vi "State Machine Air Heater Control.vi"() -> ()   [LabVIEW 2022 SP3]
uses:
  <vilib>/MakerHub/LINX/Public/Peripherals/Analog/Analog Read 1 Chan.vi
  <vilib>/MakerHub/LINX/Public/Peripherals/PWM/PWM Set Duty Cycle 1 Chan.vi
  <vilib>/MakerHub/LINX/Public/Peripherals/Analog/Analog Read N Chans.vi
  <vilib>/MakerHub/LINX/Private/Local IO/LinxAnalogRead.vi
  <vilib>/MakerHub/LINX/Public/Utilities/Check Channel.vi
  <vilib>/MakerHub/LINX/Private/Utilties/Generate Error.vi
  <vilib>/MakerHub/LINX/Public/Peripherals/PWM/PWM Set Duty Cycle N Chans.vi
  <vilib>/MakerHub/LINX/Public/Utilities/Open Serial.vi
  <vilib>/MakerHub/LINX/LMH-LINX.lvlib
panel:
  in  "Room Temp [Deg C]":dbl=25.0 format="%.1g"
  out "Count":dbl
  in  "Ts [s]":dbl=0.1
  in  "?":T1(tab)
  in  "Ti [sec]":dbl=6.0
  in  "Kp":dbl=0.35
  in  "API Key":string="8S5CEVLQ8GQW3VRW"
  in  "Channel Field":i32=1
  in  "Temperature Read Channel":dbl
  in  "PWM Channel":u8=9
  in  "Arduino Serial Port":refnum<visa-resource-name>="COM8"
  out "Control Signal [V]":dbl format="%.1g"
  in  "Temp Set Point [Deg]":dbl=35.0 format="%.1f"
  out "Temperature Chart":T2(graph)={"Filter Output"=35.087076822916664, "Temp Set Point [Deg]"=35.0}
  out "Temperature [Deg C]":dbl=25.0 format="%.1g"
  in  "Stop Button":bool
  out "Error Out":errorcluster
  in  "Error Out":errorcluster
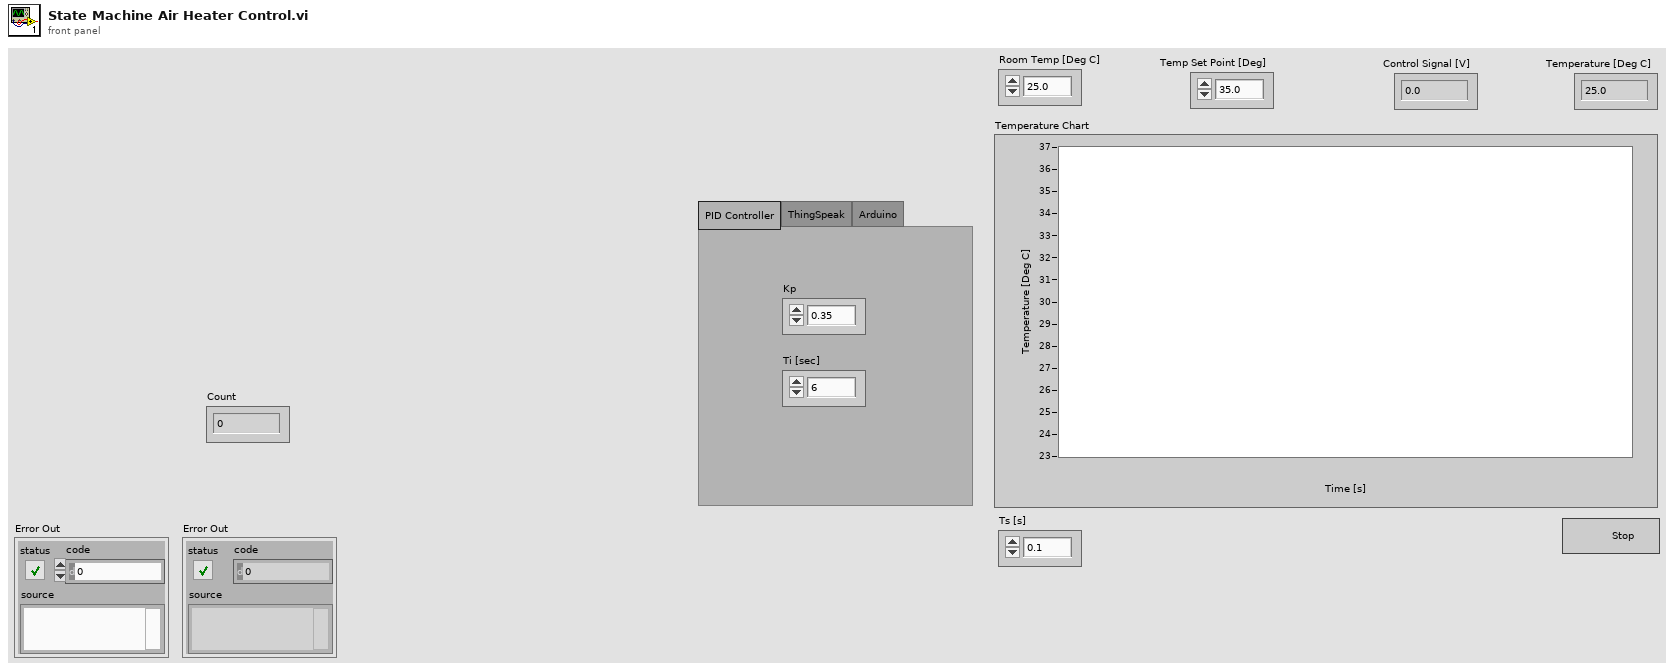
[diagram p1: front panel]
types:
  T1 = enum32{"PID Controller", "ThingSpeak", "Arduino"}
  T2 = cluster{"Filter Output":dbl, "Temp Set Point [Deg]":dbl}
  T3 = cluster{"Filter Output":dbl, "Temp Set Point [Deg]":dbl}[]
  T4 = typedef "LMH-LINX.lvlib/LINX Ref.ctl" = cluster{"IO":T5, "Interface":T6, "LINX Device Config":T7}
  T5 = typedef "LMH-LINX.lvlib/Platform.ctl" = enum16{"Remote", "Local"}
  T6 = typedef "LMH-LINX.lvlib/Interface.ctl" = enum16{"Serial", "TCP"}
  T7 = typedef "LMH-LINX.lvlib/Device.lvlib/LINX Device Config.ctl" = cluster{"Interface":T6, "COM Port":refnum<visa-resource-name>, "TCP Configuration":T8, "Device Family":u8, "Device ID":u8, "Device Name":string, "TCP Ref":refnum<k5>, "Channels":T9}
  T8 = typedef "LMH-LINX.lvlib/Device.lvlib/TCP Config.ctl" = cluster{"IP Address":string, "Port":u16}
  T9 = typedef "LMH-LINX.lvlib/Channels.ctl" = cluster{"DI":u8[], "DO":u8[], "AI":u8[], "AO":u8[], "PWM":u8[], "QE":u8[], "UART":u8[], "I2C 2":u8[], "SPI":u8[], "CAN":u8[], "Servo":u8[], "AI Ref (V)":dbl, "AI Resolution (Bits)":u8, "AO Ref (V)":dbl, "AO Resolution (Bits)":u8}
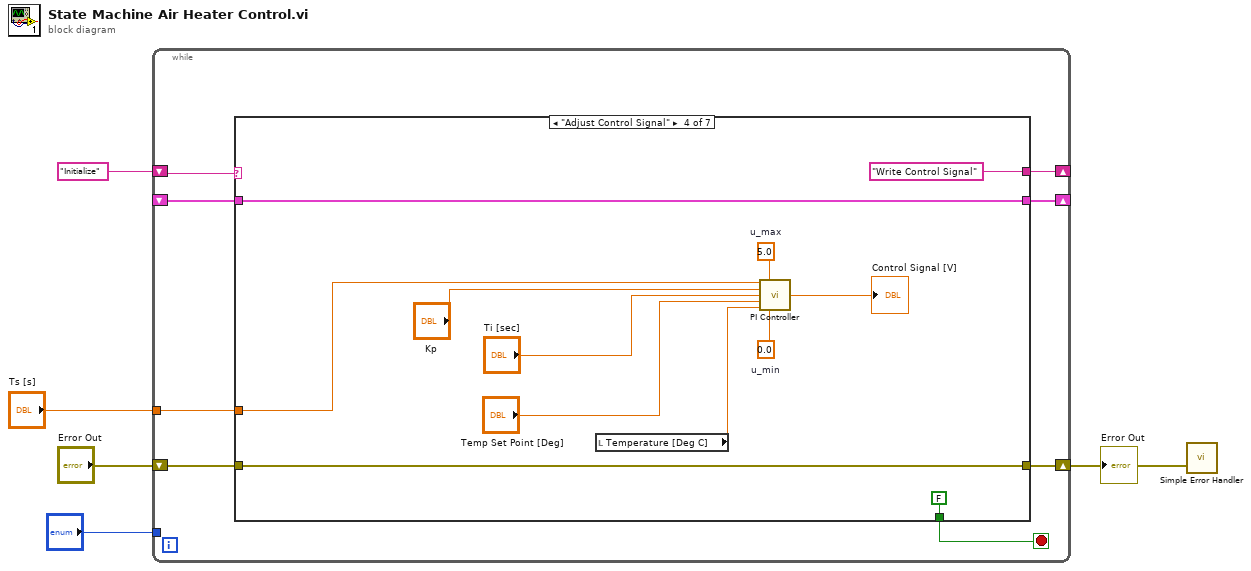
[diagram p0: block diagram]
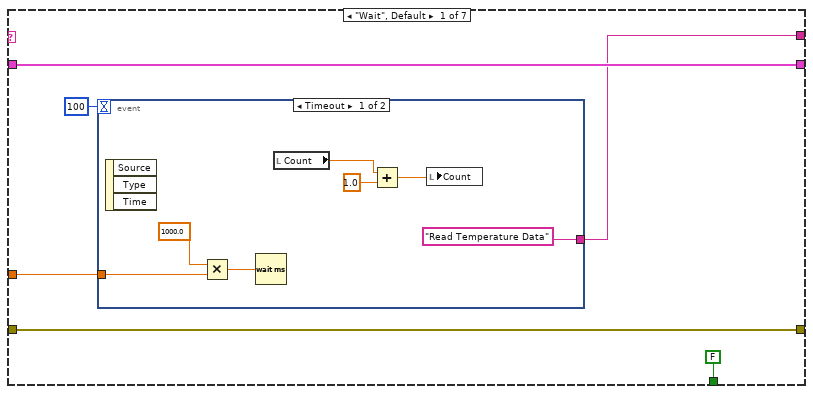
[diagram p2: hidden frame]
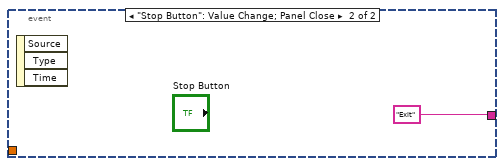
[diagram p3: hidden frame]
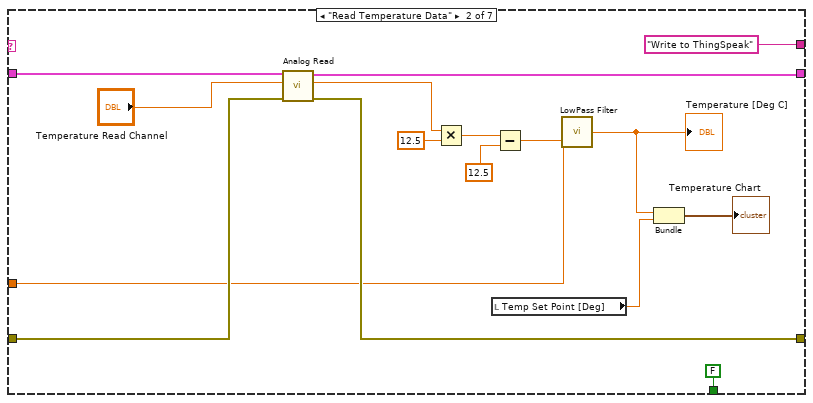
[diagram p4: hidden frame]
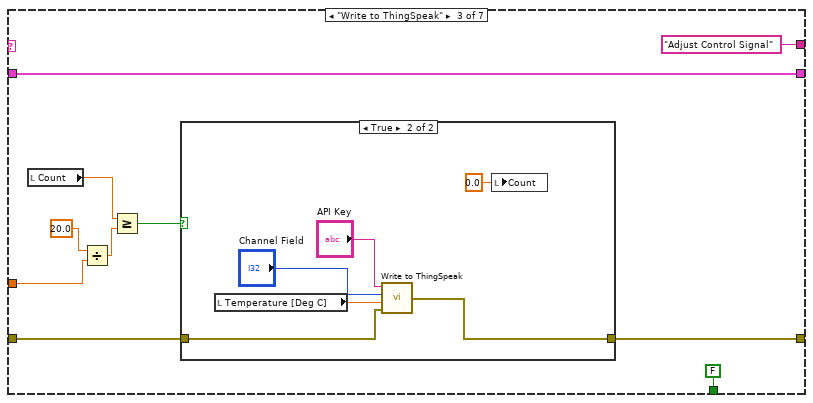
[diagram p5: hidden frame]
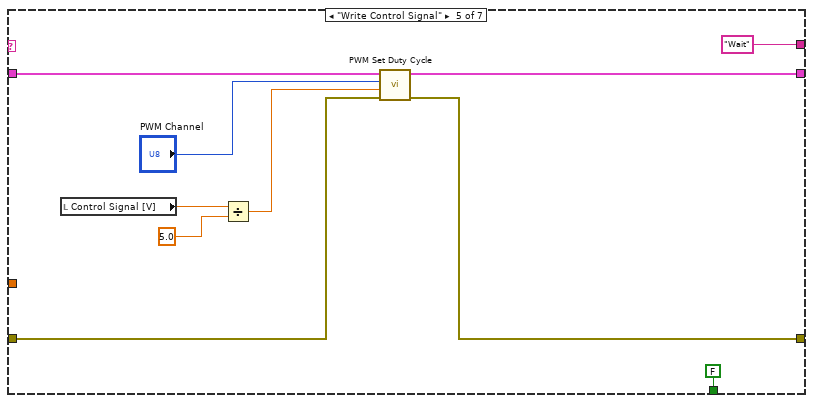
[diagram p7: hidden frame]
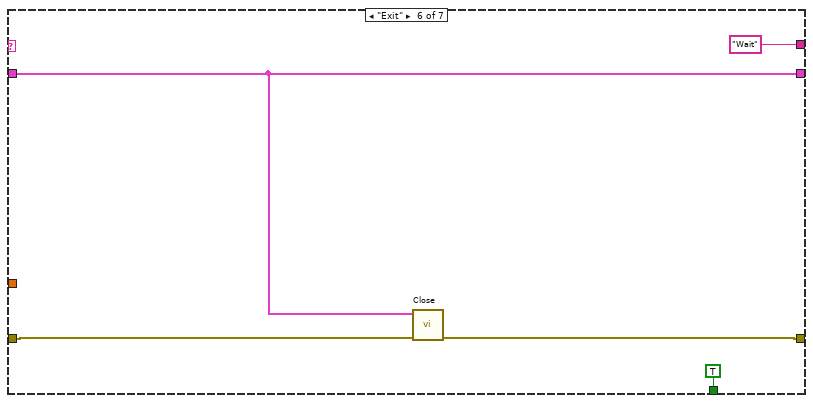
[diagram p8: hidden frame]
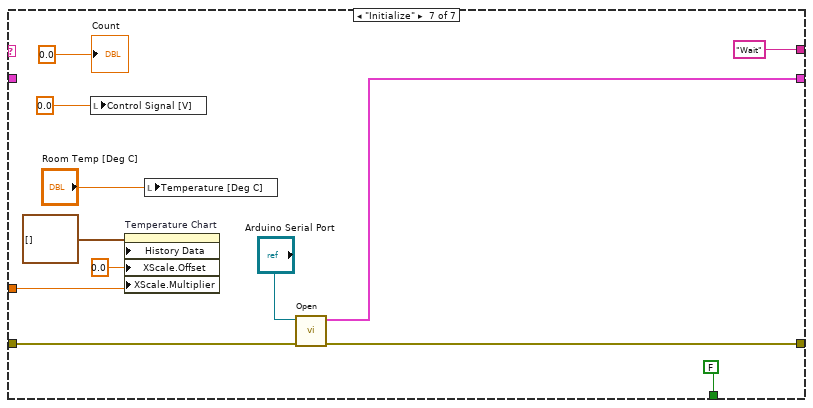
[diagram p9: hidden frame]
diagram:
  n1 = while {
    shift-right: [w8] -> _
    shift-left: "Initialize" -> [w13]
    shift-right: [w11] -> w3
    shift-left: "Error Out" -> [w12]
    shift-right: [w10] -> _
    shift-left: _ -> [w7]
    tunnel: "Ts [s]" -> [w6]
    tunnel: "?" -> [_]
    stop <- w9 stop-if-true
    n2 = case shown="\"Adjust Control Signal\"" w13 {
      tunnel: w12 -> [w18 w42 w53 w71 w79 w86 w99]
      tunnel: [w18 w41 w52 w71 w78 w85 w98] -> w11
      tunnel: [w19 w40 w51 w70 w81 w84 w96] -> w10
      tunnel: [FALSE FALSE FALSE FALSE FALSE TRUE FALSE] -> w9
      tunnel: [w16 "Write to ThingSpeak" "Adjust Control Signal" "Write Control Signal" "Wait" "Wait" "Wait"] -> w8
      tunnel: w7 -> [w19 w43 w51 w70 w82 w84 _]
      tunnel: w6 -> [w15 w34 w45 w61 _ _ w93]
      frame "Wait", Default {
        n3 = event shown="[0] Timeout" {
          selector: _ -> [_ _]
          dyn-events: _ -> [_ _]
          timeout: 100 -> [_ _]
          tunnel: ["Read Temperature Data" "Exit"] -> w16
          tunnel: w15 -> [w23 _]
          event Timeout {
            n4 = event-data() -> ()  [unwired: 1 in, 3 out]
            n5 = Multiply(x=1000.0, y=w23) -> (x*y=w25:dbl)
            n6 = Wait (ms)(milliseconds to wait=w25) -> ()  [unwired: 1 out]
            n7 = local read "Count"() -> (w22:dbl)
            n8 = Add(x=w22, y=1.0) -> (x+y=w20:dbl)
            n9 = local write "Count"(w20) -> ()
          }
          event "Stop Button": Value Change; Panel Close {
            n10 = event-data() -> ()  [unwired: 1 in, 3 out]
          }
        }
      }
      frame "Read Temperature Data" {
        n11 = call-poly <vilib>:"Analog Read.vi"("Error In"=w42, "Analog Channel"="Temperature Read Channel", "LINX Resource"=w43) -> ("Error Out"=w41:errorcluster, "Voltage"=w39:dbl, "LINX Resource"=w40:T4)  [unwired: 5 in, 1 out]
        n12 = Multiply(x=w39, y=12.5) -> (x*y=w37:dbl)
        n13 = local read "Temp Set Point [Deg]"() -> (w29:dbl)
        n14 = Subtract(x=w37, y=12.5) -> (x-y=w35:dbl)
        n15 = call "LowPass Filter.vi"("Filter Input"=w35, "Ts [s]"=w34) -> ("Filter Output"=w30:dbl)
        "Temperature [Deg C]" <- w30
        n16 = Bundle("Filter Output"=w30, "Temp Set Point [Deg]"=w29) -> (→"Temperature Chart":T2)  [unwired: 1 in]
      }
      frame "Write to ThingSpeak" {
        n17 = local read "Count"() -> (w48:dbl)
        n18 = Divide(x=20.0 ("y"), y=w45) -> (x/y=w44:dbl)
        n19 = Greater Or Equal?(x=w48, y=w44) -> (x >= y?=w47:bool)
        n20 = case shown="True" w47 {
          tunnel: w53 -> [w54 w60]
          tunnel: [w54 w59] -> w52
          frame False {
          }
          frame True {
            n21 = local read "Temperature [Deg C]"() -> (w58:dbl)
            n22 = call "Write to ThingSpeak.vi"("error in"=w60, "Temp Value"=w58, "Field"="Channel Field", "API Key"="API Key") -> ("error out"=w59:errorcluster)
            n23 = local write "Count"(0.0 ("Count")) -> ()
          }
        }
      }
      frame "Adjust Control Signal" {
        w66 = 5.0  # u_max
        w67 = 0.0  # u_min
        n24 = local read "Temperature [Deg C]"() -> (w65:dbl)
        n25 = call "PI Controller.vi"("Ts [s]"=w61, "u_max"=w66, "Kp"="Kp", "Ti [s]"="Ti [sec]", "Reference Value"="Temp Set Point [Deg]", "Process Value"=w65, "u_min"=w67) -> ("Output"=→"Control Signal [V]":dbl)  [unwired: 8 in]
      }
      frame "Write Control Signal" {
        n26 = local read "Control Signal [V]"() -> (w76:dbl)
        n27 = Divide(x=w76, y=5.0) -> (x/y=w74:dbl)
        n28 = call-poly <vilib>:"PWM Set Duty Cycle.vi"("Error In"=w79, "Duty Cycle (0-1)"=w74, "PWM Channel"="PWM Channel", "LINX Resource"=w82) -> ("Error Out"=w78:errorcluster, "LINX Resource"=w81:T4)  [unwired: 6 in]
      }
      frame "Exit" {
        n29 = call <vilib>:"Close.vi"("Error In"=w86, "LINX Resource"=w84) -> ("Error Out"=w85:errorcluster)  [unwired: 9 in]
      }
      frame "Initialize" {
        n30 = local write "Control Signal [V]"(0.0 ("Control Signal [V]")) -> ()
        n31 = property on="Temperature Chart" class="WFChart (strict)"("History Data"=T3 [], "XScale.Offset"=0.0 ("X Scale.Offset and Multiplier:Offset"), "XScale.Multiplier"=w93) -> ()  [unwired: 2 in, 2 out]
        n32 = local write "Temperature [Deg C]"("Room Temp [Deg C]") -> ()
        n33 = call-poly <vilib>:"Open.vi"("Error In"=w99, "Serial Port"="Arduino Serial Port") -> ("Error Out"=w98:errorcluster, "LINX Resource"=w96:T4)  [unwired: 7 in, 1 out]
        "Count" <- 0.0 ("Count")
      }
    }
  }
  "Error Out" <- w3
  n34 = call <vilib>:"Simple Error Handler.vi"("error in (no error)"=w3) -> ()  [unwired: 4 in, 5 out]
